vi "StutterShifterState.vi"(9 "Shifter_Mode":bool, 10 "Enable_Stutter":bool) -> (2 "New_Shifter_Mode":bool)   [LabVIEW 2019]
panel:
  in  "Stutter_Time":u32
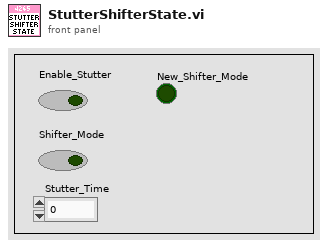
[diagram p1: front panel]
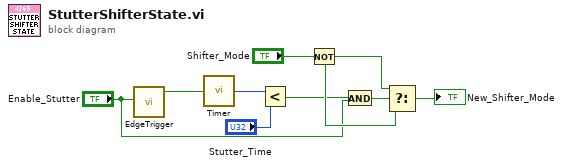
[diagram p0: block diagram]
diagram:
  n1 = call "EdgeTrigger.vi"("Input Signal"="Enable_Stutter") -> ("Rising Edge Trigger"=w9:bool)  [unwired: 2 out]
  n2 = call "Timer.vi"("Reset Timer"=w9) -> ("Time (ms)"=w8:u32)
  n3 = Less?(x=w8, y="Stutter_Time") -> (x < y?=w4:bool)
  n4 = Not(x="Shifter_Mode") -> (.not. x?=w7:bool)
  n5 = And(x=w4, y="Enable_Stutter") -> (x .and. y?=w5:bool)
  n6 = Select(t=w7, s=w5, f="Shifter_Mode") -> (s? t:f=→"New_Shifter_Mode":bool)
